vi "Test 2 Get Number Coordinates.vi"(8 "error in (no error)":errorcluster, 11 "Test Case In":refnum<class "Schema parsing test.lvclass">) -> (0 "error out":errorcluster, 3 "Test Case Out":refnum<class "Schema parsing test.lvclass">)   [LabVIEW 2020, in "Schema parsing test.lvclass"]
uses:
  Schema parsing test.lvclass
  C:/Program Files (x86)/National Instruments/LabVIEW 2020/vi.lib/Astemes/LUnit/Test Case.lvclass
  <vilib>/Astemes/LUnit/Test Case.lvclass/Test Case.ctl
  4993e8ee-a06a-463a-9684-69129f64d5ce.vi
  <vilib>/Astemes/LUnit/Append Pass Result.vi
  <vilib>/Astemes/LUnit/Append Fail Result.vi
  <vilib>/Astemes/LUnit/Describe Comparison.vi
  <vilib>/Astemes/LUnit/Compare Variants.vi
  <vilib>/Astemes/LUnit/Variant to string.vi
  <vilib>/Utility/Data Type/Get Type Information.vi
  <vilib>/Utility/LVClass/Get LV Class Name.vi
  Number/Number.lvclass
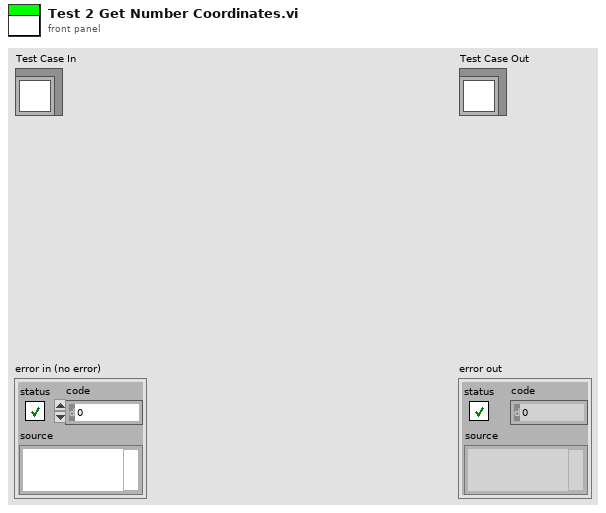
[diagram p1: front panel]
types:
  T1 = typedef "Number.lvclass/Coordinate.ctl" = cluster{"Col":i32, "Row":i32}
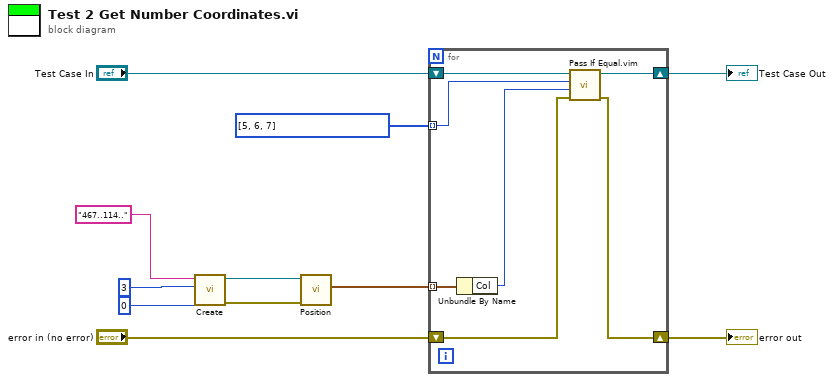
[diagram p0: block diagram]
diagram:
  n1 = call "Create.vi"("Row"=0, "Col Offset"=3, "String"="467..114..") -> ("error out"=w3:errorcluster, "Number"=w4:refnum<class "Number.lvclass">)  [unwired: 6 in, 1 out]
  n2 = call "Position.vi"("error in (no error)"=w3, "Number in"=w4) -> ("Position"=w2:T1[])  [unwired: 7 in, 2 out]
  n3 = for {
    shift-right: [w17] -> w10
    shift-left: "Test Case In" -> [w18]
    shift-right: [w15] -> w8
    shift-left: "error in (no error)" -> [w16]
    tunnel: w2 -> [w14] mode=indexing
    tunnel: i32[] [5, 6, 7] ("Col") -> [w12] mode=indexing
    n4 = Unbundle By Name(w14) -> ("Col"=w13:i32)
    n5 = call "Pass If Equal.vim"("error in (no error)"=w16, "Actual"=w13, "Expected"=w12, "LUnit Test Case In"=w18) -> ("error out"=w15:errorcluster, "LUnit Test Case Out"=w17:refnum<class "Schema parsing test.lvclass">)  [unwired: 6 in]
  }
  "error out" <- w8
  "Test Case Out" <- w10
